vi "UnitTest_1.vi"   [LabVIEW 2014, in "TableLogger_SQLite_Actor.lvlib" / "TableLogger_SQLite_Actor.lvclass"]
uses:
  TableLogger_SQLite_Actor.lvclass
  TableLogger_Actor/TableLoggerConfig.ctl
  TableLogger_Actor/TableLoggerTypes.ctl
  TableLogger_Actor/TableLoggerBackupConfig.ctl
  TableLogger_Actor/TableLogger_Actor.lvlib
types:
  T1 = cluster{"Numeric Data":i32, "Float Data":dbl, "String Data":string, "Enum Data":enum16{"Enum Item 1", "Enum Item 2"}, "Array Data":i32[], "Array Data 2":i32[]}[]
  T2 = cluster{"Numeric Data":i32, "Float Data":dbl, "String Data":string, "Enum Data":enum16{"Enum Item 1", "Enum Item 2"}, "Array Data":i32[]}
  T3 = typedef "TableLogger_Actor.lvlib/TableLoggerConfig.ctl" = cluster{"TableLogger":T4, "DB File Path":path, "DB Backup Config":T5}
  T4 = typedef "TableLogger_Actor.lvlib/TableLoggerTypes.ctl" = enum16{"CSV Logger", "SQLite Logger"}
  T5 = typedef "TableLogger_Actor.lvlib/TableLoggerBackupConfig.ctl" = cluster{"Directory":path, "UTC Time Format":bool, "On Launch":bool, "Interval (Hours)":dbl, "Size Multiples (Bytes)":i32}
  T6 = cluster{"FC Flow Set":dbl, "FM Flow Measure":dbl, "UUT Data":dbl, "Stage 1  Flow Meas":cluster{"FC Flow Set":dbl, "FM Flow Measure":dbl, "UUT Data":dbl}[]}[]
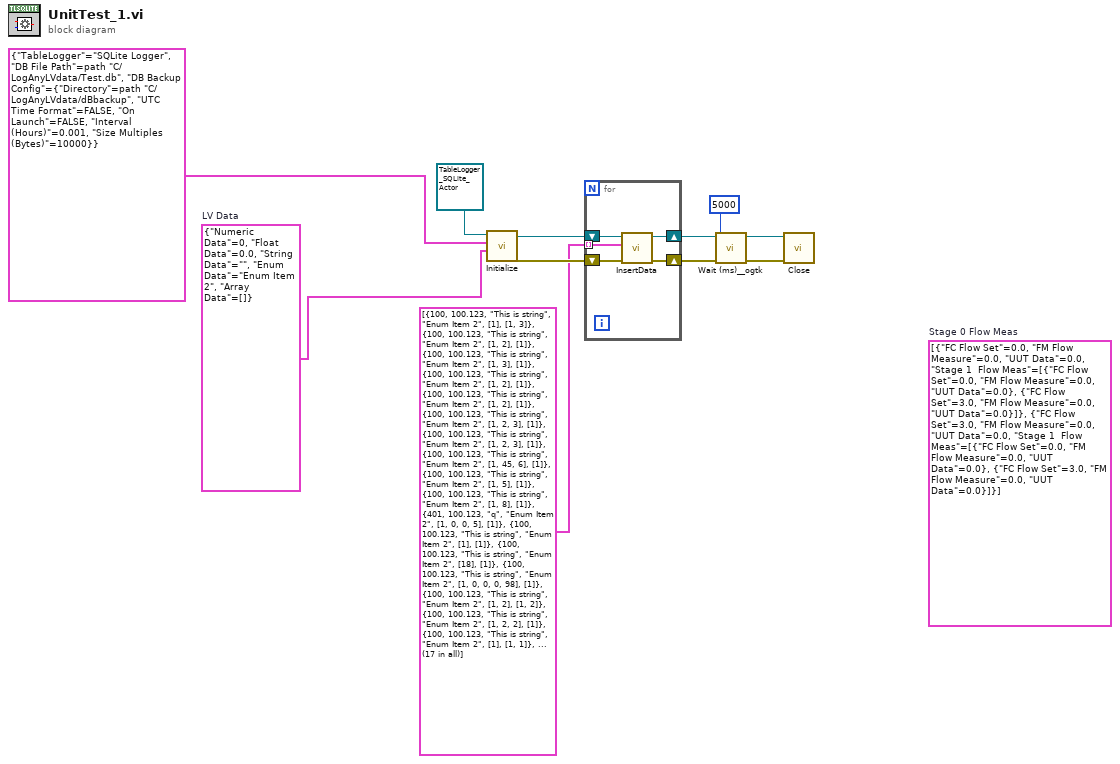
[diagram p0: block diagram]
diagram:
  w4 = T2 {"Numeric Data"=0, "Float Data"=0.0, "String Data"="", "Enum Data"=enum."Enum Item 2", "Array Data"=[]}  # LV Data
  (unwired) T6 [{"FC Flow Set"=0.0, "FM Flow Measure"=0.0, "UUT Data"=0.0, "Stage 1  Flow Meas"=[{"FC Flow Set"=0.0, "FM Flow Measure"=0.0, "UUT Data"=0.0}, {"FC Flow Set"=3.0, "FM Flow Measure"=0.0, "UUT Data"=0.0}]}, {"FC Flow Set"=3.0, "FM Flow Measure"=0.0, "UUT Data"=0.0, "Stage 1  Flow Meas"=[{"FC Flow Set"=0.0, "FM Flow Measure"=0.0, "UUT Data"=0.0}, {"FC Flow Set"=3.0, "FM Flow Measure"=0.0, "UUT Data"=0.0}]}]  # Stage 0 Flow Meas
  n1 = call-dynamic "Initialize.vi"("Data Cluster (for Table Headers)"=w4, "TableLogger Config"=T3 {"TableLogger"=enum."SQLite Logger", "DB File Path"=path "C:/LogAnyLVdata/Test.db", "DB Backup Config"={"Directory"=path "C:/LogAnyLVdata/dBbackup", "UTC Time Format"=FALSE, "On Launch"=FALSE, "Interval (Hours)"=0.001, "Size Multiples (Bytes)"=10000}}, "object in"=refnum<class "TableLogger_SQLite_Actor.lvclass"> refnum) -> ("error out"=w9:errorcluster, "object out"=w6:refnum<class "TableLogger_SQLite_Actor.lvclass">)  [unwired: 7 in]
  n2 = for {
    shift-right: [w14] -> w8
    shift-left: w9 -> [w15]
    shift-right: [w12] -> w5
    shift-left: w6 -> [w13]
    tunnel: T1 [{"Numeric Data"=100, "Float Data"=100.123, "String Data"="This is string", "Enum Data"=enum."Enum Item 2", "Array Data"=[1], "Array Data 2"=[1, 3]}, {"Numeric Data"=100, "Float Data"=100.123, "String Data"="This is string", "Enum Data"=enum."Enum Item 2", "Array Data"=[1, 2], "Array Data 2"=[1]}, {"Numeric Data"=100, "Float Data"=100.123, "String Data"="This is string", "Enum Data"=enum."Enum Item 2", "Array Data"=[1, 3], "Array Data 2"=[1]}, {"Numeric Data"=100, "Float Data"=100.123, "String Data"="This is string", "Enum Data"=enum."Enum Item 2", "Array Data"=[1, 2], "Array Data 2"=[1]}, {"Numeric Data"=100, "Float Data"=100.123, "String Data"="This is string", "Enum Data"=enum."Enum Item 2", "Array Data"=[1, 2], "Array Data 2"=[1]}, {"Numeric Data"=100, "Float Data"=100.123, "String Data"="This is string", "Enum Data"=enum."Enum Item 2", "Array Data"=[1, 2, 3], "Array Data 2"=[1]}, {"Numeric Data"=100, "Float Data"=100.123, "String Data"="This is string", "Enum Data"=enum."Enum Item 2", "Array Data"=[1, 2, 3], "Array Data 2"=[1]}, {"Numeric Data"=100, "Float Data"=100.123, "String Data"="This is string", "Enum Data"=enum."Enum Item 2", "Array Data"=[1, 45, 6], "Array Data 2"=[1]}, {"Numeric Data"=100, "Float Data"=100.123, "String Data"="This is string", "Enum Data"=enum."Enum Item 2", "Array Data"=[1, 5], "Array Data 2"=[1]}, {"Numeric Data"=100, "Float Data"=100.123, "String Data"="This is string", "Enum Data"=enum."Enum Item 2", "Array Data"=[1, 8], "Array Data 2"=[1]}, {"Numeric Data"=401, "Float Data"=100.123, "String Data"="q", "Enum Data"=enum."Enum Item 2", "Array Data"=[1, 0, 0, 5], "Array Data 2"=[1]}, {"Numeric Data"=100, "Float Data"=100.123, "String Data"="This is string", "Enum Data"=enum."Enum Item 2", "Array Data"=[1], "Array Data 2"=[1]}, {"Numeric Data"=100, "Float Data"=100.123, "String Data"="This is string", "Enum Data"=enum."Enum Item 2", "Array Data"=[18], "Array Data 2"=[1]}, {"Numeric Data"=100, "Float Data"=100.123, "String Data"="This is string", "Enum Data"=enum."Enum Item 2", "Array Data"=[1, 0, 0, 0, 98], "Array Data 2"=[1]}, {"Numeric Data"=100, "Float Data"=100.123, "String Data"="This is string", "Enum Data"=enum."Enum Item 2", "Array Data"=[1, 2], "Array Data 2"=[1, 2]}, {"Numeric Data"=100, "Float Data"=100.123, "String Data"="This is string", "Enum Data"=enum."Enum Item 2", "Array Data"=[1, 2, 2], "Array Data 2"=[1]}, {"Numeric Data"=100, "Float Data"=100.123, "String Data"="This is string", "Enum Data"=enum."Enum Item 2", "Array Data"=[1], "Array Data 2"=[1, 1]}] -> [w11] mode=indexing
    n3 = call-dynamic "InsertData.vi"("error in (no error)"=w15, "Data Cluster"=w11, "object in"=w13) -> ("error out"=w14:errorcluster, "object out"=w12:refnum<class "TableLogger_SQLite_Actor.lvclass">)  [unwired: 7 in]
  }
  n4 = call "Wait (ms)__ogtk.vi"("error in (no error)"=w8, "milliseconds to wait"=u32 5000) -> ("error out"=w2:errorcluster)  [unwired: 8 in, 1 out]
  n5 = call-dynamic "Close.vi"("error in (no error)"=w2, "object in"=w5) -> ()  [unwired: 8 in, 2 out]
